vi "Read Field (N.O.).vi"(8 "error in (no error)":errorcluster, 10 "VISA session":refnum<visa-resource-name>, 11 "input cluster":T1) -> (0 "error out":errorcluster, 1 "Current":string, 2 "Field (T)":dbl format="%_6f", 3 "output cluster":T1, 4 "Voltage":string, 5 "dup VISA session":refnum<visa-resource-name>)   [LabVIEW 2012]
uses:
  Magna Power Constants.vi
  <vilib>/gmath/NI_Gmath.lvlib
panel:
  out "Fluke Voltage (V)":dbl format="%.6f"
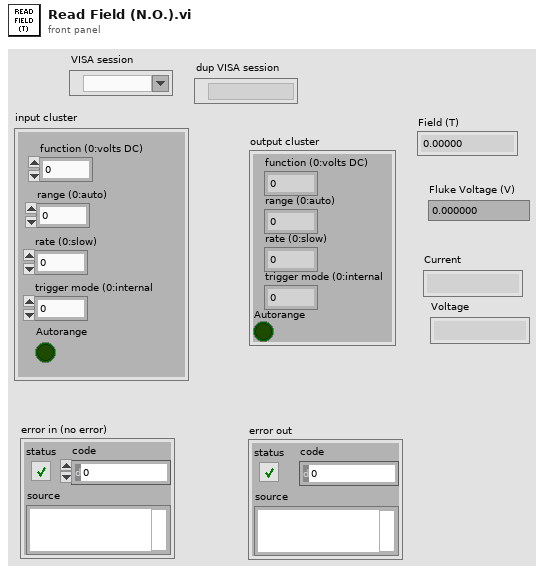
[diagram p1: front panel]
types:
  T1 = cluster{"function (0:volts DC)":i16, "range (0:auto)":i16, "rate (0:slow)":i16, "trigger mode (0:internal":i16, "Autorange":bool}
  T2 = cluster{"Magna Current":dbl[], "Magnetic Field":dbl[], "Fluke Voltage":dbl[]}
  T3 = cluster{"function (0:volts DC)":u16, "range (0:auto)":u16, "rate (0:slow)":u16, "trigger mode (0:internal)":u16, "Autorange":bool}
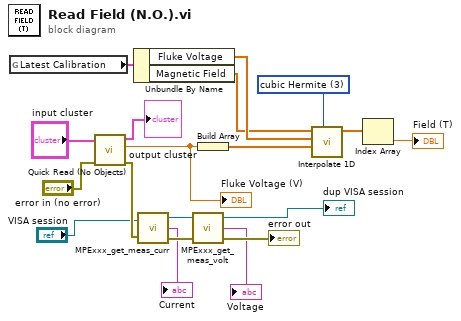
[diagram p0: block diagram]
diagram:
  w9 = 3 items=["nearest", "linear", "spline", "cubic Hermite", "Lagrange"] ("method")
  n1 = global read "Magna Power Constants.vi" "Latest Calibration"() -> (w19:T2)
  n2 = call "Quick Read (No Objects).vi"("error in (no error)"="error in (no error)", "Fluke Multimeter In"="input cluster") -> ("error out"=w8:errorcluster, "measurement"=w13:dbl, "Fluke Multimeter Out"=→"output cluster":T3)  [unwired: 6 in, 1 out]
  "Fluke Voltage (V)" <- w13
  n3 = Unbundle By Name(w19) -> ("Fluke Voltage"=w15:dbl[], "Magnetic Field"=w14:dbl[])
  n4 = call "MPExxx_get_meas_curr.vi"("VISA session"="VISA session", "error in (no error)"=w8) -> ("dup VISA session"=w3:refnum<visa-resource-name>, "Output Current"=→"Current":string, "error out"=w7:errorcluster)
  n5 = call "MPExxx_get_meas_volt.vi"("VISA session"=w3, "error in (no error)"=w7) -> ("dup VISA session"=→"dup VISA session":refnum<visa-resource-name>, "Output Voltage"=→"Voltage":string, "error out"=→"error out":errorcluster)
  n6 = Build Array(w13) -> (w12:dbl[])
  n7 = call <vilib>:"Interpolate 1D.vi"("method"=w9, "xi"=w12, "X"=w15, "Y"=w14) -> ("yi"=w11:dbl[])  [unwired: 5 in, 2 out]
  n8 = Index Array(array=w11) -> (element=→"Field (T)":dbl)  [unwired: 1 in]
